vi "Enable Sync Mask.vi"(8 "error in (no error)":errorcluster, 10 "Enable":bool, 11 "Scheduler in":refnum<class "Scheduler.lvclass">) -> (0 "error out":errorcluster, 3 "Scheduler out":refnum<class "Scheduler.lvclass">)   [LabVIEW 2020, in "TALOS.lvlib" / "Scheduler.lvlib" / "Scheduler.lvclass"]
doc: "VI for change control state between 'enabled' and 'disabled and grayed out.' This VI also resets the values in the mask whenever it is disabled."
uses:
  Scheduler.lvclass
  C:/LabVIEW Code/TALOS/talos/Father of all uServices/Father of all uServices/Father of all uServices.lvclass
  Run Utilities/TypeDefs/Synchronize FPGA Cluster.ctl
  Ancestor/Ancestor/Ancestor.lvclass/Ancestor.ctl
  Support VIs/Generate Error.vi
  FGV/Error Memory/Get Error Description.vi
  Support VIs/Get PC name.vi
  Ancestor/Ancestor/Read ID.vi
  Support VIs/Get Class Name.vi
  <vilib>/Utility/error.llb/Clear Errors.vi
  FGV/Error Memory/Error Memory Core.vi
  <vilib>/AdvancedString/Delimited String to 1D String Array.vi
  Support VIs/Circus Root Path.vi
  FGV/Error Memory/Error Crt Lvl checker.vi
  FGV/Error Memory/Error Memory Core.vi/40c8088d-b597-4017-91af-faa98e00292e.vi
  FGV/Error Memory/Error Memory Core.vi/d4a3ab98-063c-4e44-b43d-fbdcfe6c2be2.vi
  Support VIs/Global Memory.vi
  <vilib>/Utility/LVClass/Get LV Class Name.vi
  Support VIs/Is in Packed Library.vi
  Support VIs/TALOS Root path.vi
  Support VIs/Read CSV worksheet.vi
  Support VIs/Global Constants.vi
  <vilib>/Utility/error.llb/General Error Handler.vi
  Support VIs/Error Log.vi
  Ancestor/Ancestor/Ancestor.lvclass
  <vilib>/Comparison/Equal/Equal Functor/Equal Functor.lvclass
  Father of all uServices/Father of all uServices/Father of all uServices.lvclass
  TALOS.lvlib
  Run Utilities/Run Utilities.lvlib
panel:
  in  "Sync. mask - template":T1[](array[typedef])
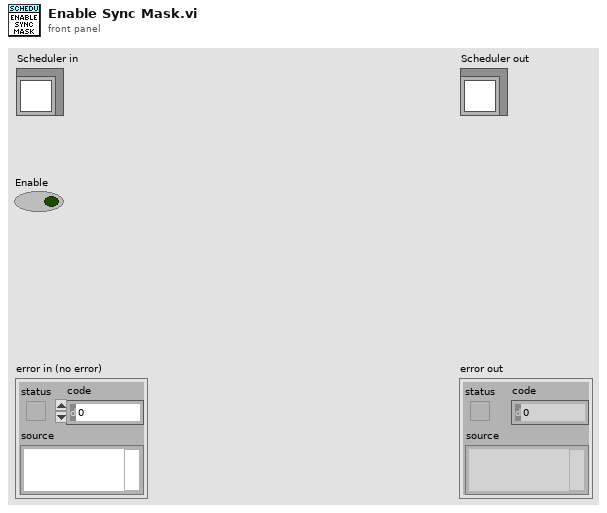
[diagram p1: front panel]
types:
  T1 = typedef "TALOS.lvlib/Run Utilities.lvlib/Synchronize FPGA Cluster.ctl" = cluster{"Status":bool, "FPGA Name":string}
  T2 = enum8{"Enabled", "Disabled", "Disabled and Grayed Out"}
  T3 = typedef "TALOS.lvlib/Run Utilities.lvlib/Synchronize Kasli Cluster.ctl" = cluster{"Status":bool, "FPGA Name":string}
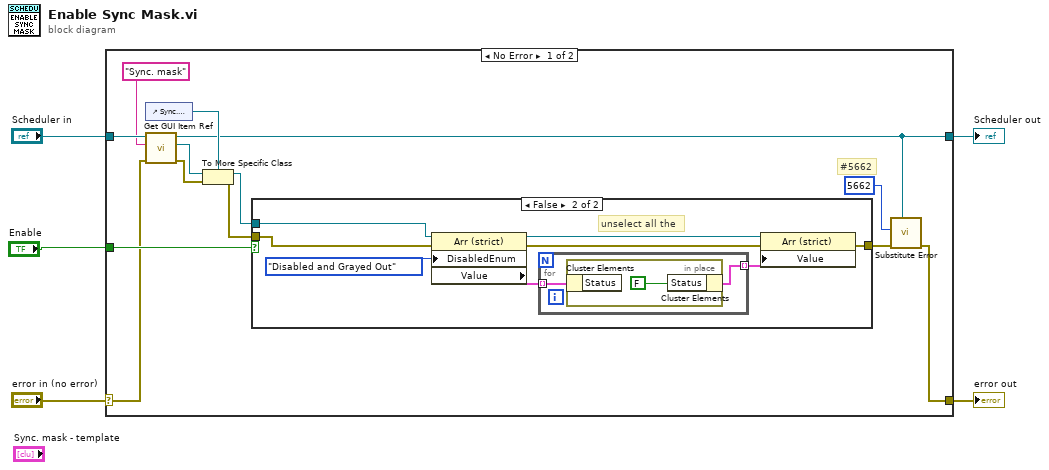
[diagram p0: block diagram]
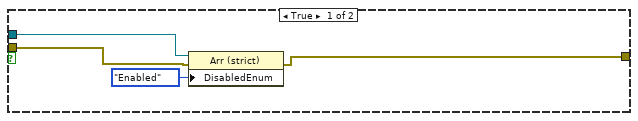
[diagram p2: hidden frame]
diagram:
  n1 = case shown="No Error" "error in (no error)" {
    selector: "error in (no error)" -> [w15 w35]
    tunnel: [w8 w35] -> w4
    tunnel: [w7 w34] -> w2
    tunnel: "Scheduler in" -> [w17 w34]
    tunnel: "Enable" -> [w18 _]
    frame No Error {
      # "#5662"
      n2 = control-ref of="Sync. mask - template"() -> (w10:refnum<vi>)
      n3 = call "Get GUI Item Ref.vi"("error in (no error)"=w15, "FP Item Name"="Sync. mask", "uService Template in"=w17) -> ("error out"=w12:errorcluster, "Ctl Refnum"=w14:refnum<vi>, "uService Template out"=w7:refnum<class "Scheduler.lvclass">)  [unwired: 6 in]
      n4 = To More Specific Class(target class=w10, reference=w14, error in=w12) -> (specific class reference=w13:refnum<vi>, error out=w11:errorcluster)
      n5 = case shown="False" w18 {
        tunnel: w13 -> [w21 w24]
        tunnel: w11 -> [w19 w26]
        tunnel: [w20 w23] -> w9
        frame True {
          n6 = property class="Arr (strict)"(reference=w21, error in=w19, "DisabledEnum"=T2."Enabled" ("Disabled")) -> (error out=w20:errorcluster)  [unwired: 1 out]
        }
        frame False {
          # "unselect all the"
          n7 = property class="Arr (strict)"(reference=w24, error in=w26, "DisabledEnum"=T2."Disabled and Grayed Out" ("Disabled")) -> (reference out=w27:refnum<vi>, error out=w25:errorcluster, "Value"=w29:T3[])
          n8 = for {
            tunnel: w29 -> [w32] mode=indexing
            tunnel: [w31] -> w28 mode=indexing
            n9 = in-place {
              n10 = in-place-cluster #1(w32) -> ()  [unwired: 1 out]
              n11 = in-place-cluster #1("Status"=FALSE) -> (w31:T3)
            }
          }
          n12 = property class="Arr (strict)"(reference=w27, error in=w25, "Value"=w28) -> (error out=w23:errorcluster)  [unwired: 1 out]
        }
      }
      n13 = call "Substitute Error.vi"("LabVIEW Object"=w7, "error in (no error)"=w9, "Error Code"=5662) -> ("error out"=w8:errorcluster)  [unwired: 8 in]
    }
    frame Error {
    }
  }
  "error out" <- w4
  "Scheduler out" <- w2
